vi "VISJS Viewer.vi"(4 "Extra Scripts":string, 5 "FileDependency out":map{path, T1}(c390), 6 "Options":string, 7 "OpenWebBrowser(False)":bool, 8 "error in":errorcluster, 9 "Embedd VISJS Librarya in HTMl File(False)":bool, 10 "HTMLFilePath":path, 11 "LibraryDependency":map{path, T3}(c390)) -> (0 "error out":errorcluster, 3 "HTMLFileContent":string)   [LabVIEW 2020, in "VISJS Viewer.lvlib"] (continued)
this.evTarget,this.domHandler),this.evWin&&Bp(Sp(this.element),this.evWin,this.domHandler)},t.destroy=function(){this.evEl&&zp(this.element,this.evEl,this.domHandler),this.evTarget&&zp(this.target,this.evTarget,this.domHandler),this.evWin&&zp(Sp(this.element),this.evWin,this.domHandler)},g}();function Fp(g,t,A){if(g.indexOf&&!A)return g.indexOf(t);for(var e=0;e<g.length;){if(A&&g[e][A]==t||!A&&g[e]===t)return e;e++}return-1}var Gp={pointerdown:op,pointermove:2,pointerup:np,pointercancel:rp,pointerout:rp},jp={2:Cp,3:\"pen\",4:Ip,5:\"kinect\"},Lp=\"pointerdown\",Vp=\"pointermove pointerup pointercancel\";Fu.MSPointerEvent&&!Fu.PointerEvent&&(Lp=\"MSPointerDown\",Vp=\"MSPointerMove MSPointerUp MSPointerCancel\");var Yp=function(g){function t(){var A,e=t.prototype;return e.evEl=Lp,e.evWin=Vp,(A=g.apply(this,arguments)||this).store=A.manager.session.pointerEvents=[],A}return Su(t,g),t.prototype.handler=function(g){var t=this.store,A=!1,e=g.type.toLowerCase().replace(\"ms\",\"\"),C=Gp[e],I=jp[g.pointerType]||g.pointerType,i=I===Cp,o=Fp(t,g.pointerId,\"pointerId\");C&op&&(0===g.button||i)?o<0&&(t.push(g),o=t.length-1):C&(np|rp)&&(A=!0),o<0||(t[o]=g,this.callback(this.manager,C,{pointers:t,changedPointers:[g],pointerType:I,srcEvent:g}),A&&t.splice(o,1))},t}(Zp);function Wp(g){return Array.prototype.slice.call(g,0)}function Qp(g,t,A){for(var e=[],C=[],I=0;I<g.length;){var i=t?g[I][t]:g[I];Fp(C,i)<0&&e.push(g[I]),C[I]=i,I++}return A&&(e=t?e.sort((function(g,A){return g[t]>A[t]})):e.sort()),e}var Up={touchstart:op,touchmove:2,touchend:np,touchcancel:rp},_p=function(g){function t(){var A;return t.prototype.evTarget=\"touchstart touchmove touchend touchcancel\",(A=g.apply(this,arguments)||this).targetIds={},A}return Su(t,g),t.prototype.handler=function(g){var t=Up[g.type],A=Kp.call(this,g,t);A&&this.callback(this.manager,t,{pointers:A[0],changedPointers:A[1],pointerType:Cp,srcEvent:g})},t}(Zp);function Kp(g,t){var A,e,C=Wp(g.touches),I=this.targetIds;if(t&(2|op)&&1===C.length)return I[C[0].identifier]=!0,[C,C];var i=Wp(g.changedTouches),o=[],n=this.target;if(e=C.filter((function(g){return kp(g.target,n)})),t===op)for(A=0;A<e.length;)I[e[A].identifier]=!0,A++;for(A=0;A<i.length;)I[i[A].identifier]&&o.push(i[A]),t&(np|rp)&&delete I[i[A].identifier],A++;return o.length?[Qp(e.concat(o),\"identifier\",!0),o]:void 0}var Hp={mousedown:op,mousemove:2,mouseup:np},Xp=function(g){function t(){var A,e=t.prototype;return e.evEl=\"mousedown\",e.evWin=\"mousemove mouseup\",(A=g.apply(this,arguments)||this).pressed=!1,A}return Su(t,g),t.prototype.handler=function(g){var t=Hp[g.type];t&op&&0===g.button&&(this.pressed=!0),2&t&&1!==g.which&&(t=np),this.pressed&&(t&np&&(this.pressed=!1),this.callback(this.manager,t,{pointers:[g],changedPointers:[g],pointerType:Ip,srcEvent:g}))},t}(Zp),Jp=2500;function qp(g){var t=g.changedPointers[0];if(t.identifier===this.primaryTouch){var A={x:t.clientX,y:t.clientY},e=this.lastTouches;this.lastTouches.push(A);setTimeout((function(){var g=e.indexOf(A);g>-1&&e.splice(g,1)}),Jp)}}function $p(g,t){g&op?(this.primaryTouch=t.changedPointers[0].identifier,qp.call(this,t)):g&(np|rp)&&qp.call(this,t)}function gf(g){for(var t=g.srcEvent.clientX,A=g.srcEvent.clientY,e=0;e<this.lastTouches.length;e++){var C=this.lastTouches[e],I=Math.abs(t-C.x),i=Math.abs(A-C.y);if(I<=25&&i<=25)return!0}return!1}var tf=function(){return function(g){function t(t,A){var e;return(e=g.call(this,t,A)||this).handler=function(g,t,A){var C=A.pointerType===Cp,I=A.pointerType===Ip;if(!(I&&A.sourceCapabilities&&A.sourceCapabilities.firesTouchEvents)){if(C)$p.call(Zu(Zu(e)),t,A);else if(I&&gf.call(Zu(Zu(e)),A))return;e.callback(g,t,A)}},e.touch=new _p(e.manager,e.handler),e.mouse=new Xp(e.manager,e.handler),e.primaryTouch=null,e.lastTouches=[],e}return Su(t,g),t.prototype.destroy=function(){this.touch.destroy(),this.mouse.destroy()},t}(Zp)}();function Af(g,t,A){return!!Array.isArray(g)&&(yp(g,A[t],A),!0)}var ef=32,Cf=1;function If(g,t){var A=t.manager;return A?A.get(g):g}function of(g){return 16&g?\"cancel\":8&g?\"end\":4&g?\"move\":2&g?\"start\":\"\"}var nf=function(){function g(g){void 0===g&&(g={}),this.options=zu({enable:!0},g),this.id=Cf++,this.manager=null,this.state=1,this.simultaneous={},this.requireFail=[]}var t=g.prototype;return t.set=function(g){return Gu(this.options,g),this.manager&&this.manager.touchAction.update(),this},t.recognizeWith=function(g){if(Af(g,\"recognizeWith\",this))return this;var t=this.simultaneous;return t[(g=If(g,this)).id]||(t[g.id]=g,g.recognizeWith(this)),this},t.dropRecognizeWith=function(g){return Af(g,\"dropRecognizeWith\",this)||(g=If(g,this),delete this.simultaneous[g.id]),this},t.requireFailure=function(g){if(Af(g,\"requireFailure\",this))return this;var t=this.requireFail;return-1===Fp(t,g=If(g,this))&&(t.push(g),g.requireFailure(this)),this},t.dropRequireFailure=function(g){if(Af(g,\"dropRequireFailure\",this))return this;g=If(g,this);var t=Fp(this.requireFail,g);return t>-1&&this.requireFail.splice(t,1),this},t.hasRequireFailures=function(){return this.requireFail.length>0},t.canRecognizeWith=function(g){return!!this.simultaneous[g.id]},t.emit=function(g){var t=this,A=this.state;function e(A){t.manager.emit(A,g)}A<8&&e(t.options.event+of(A)),e(t.options.event),g.additionalEvent&&e(g.additionalEvent),A>=8&&e(t.options.event+of(A))},t.tryEmit=function(g){if(this.canEmit())return this.emit(g);this.state=ef},t.canEmit=function(){for(var g=0;g<this.requireFail.length;){if(!(33&this.requireFail[g].state))return!1;g++}return!0},t.recognize=function(g){var t=Gu({},g);if(!mp(this.options.enable,[this,t]))return this.reset(),void(this.state=ef);56&this.state&&(this.state=1),this.state=this.process(t),30&this.state&&this.tryEmit(t)},t.process=function(g){},t.getTouchAction=function(){},t.reset=function(){},g}(),rf=function(g){function t(t){var A;return void 0===t&&(t={}),(A=g.call(this,zu({event:\"tap\",pointers:1,taps:1,interval:300,time:250,threshold:9,posThreshold:10},t))||this).pTime=!1,A.pCenter=!1,A._timer=null,A._input=null,A.count=0,A}Su(t,g);var A=t.prototype;return A.getTouchAction=function(){return[Xu]},A.process=function(g){var t=this,A=this.options,e=g.pointers.length===A.pointers,C=g.distance<A.threshold,I=g.deltaTime<A.time;if(this.reset(),g.eventType&op&&0===this.count)return this.failTimeout();if(C&&I&&e){if(g.eventType!==np)return this.failTimeout();var i=!this.pTime||g.timeStamp-this.pTime<A.interval,o=!this.pCenter||Op(this.pCenter,g.center)<A.posThreshold;if(this.pTime=g.timeStamp,this.pCenter=g.center,o&&i?this.count+=1:this.count=1,this._input=g,0===this.count%A.taps)return this.hasRequireFailures()?(this._timer=setTimeout((function(){t.state=8,t.tryEmit()}),A.interval),2):8}return ef},A.failTimeout=function(){var g=this;return this._timer=setTimeout((function(){g.state=ef}),this.options.interval),ef},A.reset=function(){clearTimeout(this._timer)},A.emit=function(){8===this.state&&(this._input.tapCount=this.count,this.manager.emit(this.options.event,this._input))},t}(nf),sf=function(g){function t(t){return void 0===t&&(t={}),g.call(this,zu({pointers:1},t))||this}Su(t,g);var A=t.prototype;return A.attrTest=function(g){var t=this.options.pointers;return 0===t||g.pointers.length===t},A.process=function(g){var t=this.state,A=g.eventType,e=6&t,C=this.attrTest(g);return e&&(A&rp||!C)?16|t:e||C?A&np?8|t:2&t?4|t:2:ef},t}(nf);function af(g){return g===lp?\"down\":g===hp?\"up\":g===ap?\"left\":g===dp?\"right\":\"\"}var df=function(g){function t(t){var A;return void 0===t&&(t={}),(A=g.call(this,zu({event:\"pan\",threshold:10,pointers:1,direction:pp},t))||this).pX=null,A.pY=null,A}Su(t,g);var A=t.prototype;return A.getTouchAction=function(){var g=this.options.direction,t=[];return g&cp&&t.push($u),g&up&&t.push(qu),t},A.directionTest=function(g){var t=this.options,A=!0,e=g.distance,C=g.direction,I=g.deltaX,i=g.deltaY;return C&t.direction||(t.direction&cp?(C=0===I?sp:I<0?ap:dp,A=I!==this.pX,e=Math.abs(g.deltaX)):(C=0===i?sp:i<0?hp:lp,A=i!==this.pY,e=Math.abs(g.deltaY))),g.direction=C,A&&e>t.threshold&&C&t.direction},A.attrTest=function(g){return sf.prototype.attrTest.call(this,g)&&(2&this.state||!(2&this.state)&&this.directionTest(g))},A.emit=function(t){this.pX=t.deltaX,this.pY=t.deltaY;var A=af(t.direction);A&&(t.additionalEvent=this.options.event+A),g.prototype.emit.call(this,t)},t}(sf),hf=function(g){function t(t){return void 0===t&&(t={}),g.call(this,zu({event:\"swipe\",threshold:10,velocity:.3,direction:cp|up,pointers:1},t))||this}Su(t,g);var A=t.prototype;return A.getTouchAction=function(){return df.prototype.getTouchAction.call(this)},A.attrTest=function(t){var A,e=this.options.direction;return e&(cp|up)?A=t.overallVelocity:e&cp?A=t.overallVelocityX:e&up&&(A=t.overallVelocityY),g.prototype.attrTest.call(this,t)&&e&t.offsetDirection&&t.distance>this.options.threshold&&t.maxPointers===this.options.pointers&&Yu(A)>this.options.velocity&&t.eventType&np},A.emit=function(g){var t=af(g.offsetDirection);t&&this.manager.emit(this.options.event+t,g),this.manager.emit(this.options.event,g)},t}(sf),lf=function(g){function t(t){return void 0===t&&(t={}),g.call(this,zu({event:\"pinch\",threshold:0,pointers:2},t))||this}Su(t,g);var A=t.prototype;return A.getTouchAction=function(){return[Ju]},A.attrTest=function(t){return g.prototype.attrTest.call(this,t)&&(Math.abs(t.scale-1)>this.options.threshold||2&this.state)},A.emit=function(t){if(1!==t.scale){var A=t.scale<1?\"in\":\"out\";t.additionalEvent=this.options.event+A}g.prototype.emit.call(this,t)},t}(sf),cf=function(g){function t(t){return void 0===t&&(t={}),g.call(this,zu({event:\"rotate\",threshold:0,pointers:2},t))||this}Su(t,g);var A=t.prototype;return A.getTouchAction=function(){return[Ju]},A.attrTest=function(t){return g.prototype.attrTest.call(this,t)&&(Math.abs(t.rotation)>this.options.threshold||2&this.state)},t}(sf),uf=function(g){function t(t){var A;return void 0===t&&(t={}),(A=g.call(this,zu({event:\"press\",pointers:1,time:251,threshold:9},t))||this)._timer=null,A._input=null,A}Su(t,g);var A=t.prototype;return A.getTouchAction=function(){return[Hu]},A.process=function(g){var t=this,A=this.options,e=g.pointers.length===A.pointers,C=g.distance<A.threshold,I=g.deltaTime>A.time;if(this._input=g,!C||!e||g.eventType&(np|rp)&&!I)this.reset();else if(g.eventType&op)this.reset(),this._timer=setTimeout((function(){t.state=8,t.tryEmit()}),A.time);else if(g.eventType&np)return 8;return ef},A.reset=function(){clearTimeout(this._timer)},A.emit=function(g){8===this.state&&(g&&g.eventType&np?this.manager.emit(this.options.event+\"up\",g):(this._input.timeStamp=Wu(),this.manager.emit(this.options.event,this._input)))},t}(nf),pf={domEvents:!1,touchAction:Ku,enable:!0,inputTarget:null,inputClass:null,cssProps:{userSelect:\"none\",touchSelect:\"none\",touchCallout:\"none\",contentZooming:\"none\",userDrag:\"none\",tapHighlightColor:\"rgba(0,0,0,0)\"}},ff=[[cf,{enable:!1}],[lf,{enable:!1},[\"rotate\"]],[hf,{direction:cp}],[df,{direction:cp},[\"swipe\"]],[rf],[rf,{event:\"doubletap\",taps:2},[\"tap\"]],[uf]];function vf(g,t){var A,e=g.element;e.style&&(yp(g.options.cssProps,(function(C,I){A=Qu(e.style,I),t?(g.oldCssProps[A]=e.style[A],e.style[A]=C):e.style[A]=g.oldCssProps[A]||\"\"})),t||(g.oldCssProps={}))}var yf=function(){function g(g,t){var A,e=this;this.options=Gu({},pf,t||{}),this.options.inputTarget=this.options.inputTarget||g,this.handlers={},this.session={},this.recognizers=[],this.oldCssProps={},this.element=g,this.input=new((A=this).options.inputClass||(Ap?Yp:ep?_p:tp?tf:Xp))(A,Pp),this.touchAction=new wp(this,this.options.touchAction),vf(this,!0),yp(this.options.recognizers,(function(g){var t=e.add(new g[0](g[1]));g[2]&&t.recognizeWith(g[2]),g[3]&&t.requireFailure(g[3])}),this)}var t=g.prototype;return t.set=function(g){return Gu(this.options,g),g.touchAction&&this.touchAction.update(),g.inputTarget&&(this.input.destroy(),this.input.target=g.inputTarget,this.input.init()),this},t.stop=function(g){this.session.stopped=g?2:1},t.recognize=function(g){var t=this.session;if(!t.stopped){var A;this.touchAction.preventDefaults(g);var e=this.recognizers,C=t.curRecognizer;(!C||C&&8&C.state)&&(t.curRecognizer=null,C=null);for(var I=0;I<e.length;)A=e[I],2===t.stopped||C&&A!==C&&!A.canRecognizeWith(C)?A.reset():A.recognize(g),!C&&14&A.state&&(t.curRecognizer=A,C=A),I++}},t.get=function(g){if(g instanceof nf)return g;for(var t=this.recognizers,A=0;A<t.length;A++)if(t[A].options.event===g)return t[A];return null},t.add=function(g){if(Af(g,\"add\",this))return this;var t=this.get(g.options.event);return t&&this.remove(t),this.recognizers.push(g),g.manager=this,this.touchAction.update(),g},t.remove=function(g){if(Af(g,\"remove\",this))return this;var t=this.get(g);if(g){var A=this.recognizers,e=Fp(A,t);-1!==e&&(A.splice(e,1),this.touchAction.update())}return this},t.on=function(g,t){if(void 0===g||void 0===t)return this;var A=this.handlers;return yp(Mp(g),(function(g){A[g]=A[g]||[],A[g].push(t)})),this},t.off=function(g,t){if(void 0===g)return this;var A=this.handlers;return yp(Mp(g),(function(g){t?A[g]&&A[g].splice(Fp(A[g],t),1):delete A[g]})),this},t.emit=function(g,t){this.options.domEvents&&function(g,t){var A=document.createEvent(\"Event\");A.initEvent(g,!0,!0),A.gesture=t,t.target.dispatchEvent(A)}(g,t);var A=this.handlers[g]&&this.handlers[g].slice();if(A&&A.length){t.type=g,t.preventDefault=function(){t.srcEvent.preventDefault()};for(var e=0;e<A.length;)A[e](t),e++}},t.destroy=function(){this.element&&vf(this,!1),this.handlers={},this.session={},this.input.destroy(),this.element=null},g}(),mf={touchstart:op,touchmove:2,touchend:np,touchcancel:rp},bf=function(g){function t(){var A,e=t.prototype;return e.evTarget=\"touchstart\",e.evWin=\"touchstart touchmove touchend touchcancel\",(A=g.apply(this,arguments)||this).started=!1,A}return Su(t,g),t.prototype.handler=function(g){var t=mf[g.type];if(t===op&&(this.started=!0),this.started){var A=wf.call(this,g,t);t&(np|rp)&&A[0].length-A[1].length==0&&(this.started=!1),this.callback(this.manager,t,{pointers:A[0],changedPointers:A[1],pointerType:Cp,srcEvent:g})}},t}(Zp);function wf(g,t){var A=Wp(g.touches),e=Wp(g.changedTouches);return t&(np|rp)&&(A=Qp(A.concat(e),\"identifier\",!0)),[A,e]}function kf(g,t,A){var e=\"DEPRECATED METHOD: \"+t+\"\\n\"+A+\" AT \\n\";return function(){var t=new Error(\"get-stack-trace\"),A=t&&t.stack?t.stack.replace(/^[^\\(]+?[\\n$]/gm,\"\").replace(/^\\s+at\\s+/gm,\"\").replace(/^Object.<anonymous>\\s*\\(/gm,\"{anonymous}()@\"):\"Unknown Stack Trace\",C=window.console&&(window.console.warn||window.console.log);return C&&C.call(window.console,e,A),g.apply(this,arguments)}}var xf=kf((function(g,t,A){for(var e=Object.keys(t),C=0;C<e.length;)(!A||A&&void 0===g[e[C]])&&(g[e[C]]=t[e[C]]),C++;return g}),\"extend\",\"Use `assign`.\"),Ef=kf((function(g,t){return xf(g,t,!0)}),\"merge\",\"Use `assign`.\");function Of(g,t,A){var e,C=t.prototype;(e=g.prototype=Object.create(C)).constructor=g,e._super=C,A&&Gu(e,A)}function Tf(g,t){return function(){return g.apply(t,arguments)}}var Df=function(){var g=function(g,t){return void 0===t&&(t={}),new yf(g,zu({recognizers:ff.concat()},t))};return g.VERSION=\"2.0.17-rc\",g.DIRECTION_ALL=pp,g.DIRECTION_DOWN=lp,g.DIRECTION_LEFT=ap,g.DIRECTION_RIGHT=dp,g.DIRECTION_UP=hp,g.DIRECTION_HORIZONTAL=cp,g.DIRECTION_VERTICAL=up,g.DIRECTION_NONE=sp,g.DIRECTION_DOWN=lp,g.INPUT_START=op,g.INPUT_MOVE=2,g.INPUT_END=np,g.INPUT_CANCEL=rp,g.STATE_POSSIBLE=1,g.STATE_BEGAN=2,g.STATE_CHANGED=4,g.STATE_ENDED=8,g.STATE_RECOGNIZED=8,g.STATE_CANCELLED=16,g.STATE_FAILED=ef,g.Manager=yf,g.Input=Zp,g.TouchAction=wp,g.TouchInput=_p,g.MouseInput=Xp,g.PointerEventInput=Yp,g.TouchMouseInput=tf,g.SingleTouchInput=bf,g.Recognizer=nf,g.AttrRecognizer=sf,g.Tap=rf,g.Pan=df,g.Swipe=hf,g.Pinch=lf,g.Rotate=cf,g.Press=uf,g.on=Bp,g.off=zp,g.each=yp,g.merge=Ef,g.extend=xf,g.bindFn=Tf,g.assign=Gu,g.inherit=Of,g.bindFn=Tf,g.prefixed=Qu,g.toArray=Wp,g.inArray=Fp,g.uniqueArray=Qp,g.splitStr=Mp,g.boolOrFn=mp,g.hasParent=kp,g.addEventListeners=Bp,g.removeEventListeners=zp,g.defaults=Gu({},pf,{preset:ff}),g}();Df.defaults;var Nf=Df;function Rf(g,t){var A=void 0!==uh&&ln(g)||g[\"@@iterator\"];if(!A){if(Rh(g)||(A=function(g,t){var A;if(!g)return;if(\"string\"==typeof g)return Pf(g,t);var e=wh(A=Object.prototype.toString.call(g)).call(A,8,-1);\"Object\"===e&&g.constructor&&(e=g.constructor.name);if(\"Map\"===e||\"Set\"===e)return Uo(g);if(\"Arguments\"===e||/^(?:Ui|I)nt(?:8|16|32)(?:Clamped)?Array$/.test(e))return Pf(g,t)}(g))||t&&g&&\"number\"==typeof g.length){A&&(g=A);var e=0,C=function(){};return{s:C,n:function(){return e>=g.length?{done:!0}:{done:!1,value:g[e++]}},e:function(g){throw g},f:C}}throw new TypeError(\"Invalid attempt to iterate non-iterable instance.\\nIn order to be iterable, non-array objects must have a [Symbol.iterator]() method.\")}var I,i=!0,o=!1;return{s:function(){A=A.call(g)},n:function(){var g=A.next();return i=g.done,g},e:function(g){o=!0,I=g},f:function(){try{i||null==A.return||A.return()}finally{if(o)throw I}}}}function Pf(g,t){(null==t||t>g.length)&&(t=g.length);for(var A=0,e=new Array(t);A<t;A++)e[A]=g[A];return e}var Mf=uh(\"DELETE\");function Bf(){var g=zf.apply(void 0,arguments);return Zf(g),g}function zf(){for(var g=arguments.length,t=new Array(g),A=0;A<g;A++)t[A]=arguments[A];if(t.length<2)return t[0];var e;if(t.length>2)return zf.apply(void 0,bh(e=[Bf(t[0],t[1])]).call(e,ch(wh(t).call(t,2))));var C=t[0],I=t[1];if(C instanceof Date&&I instanceof Date)return C.setTime(I.getTime()),C;var i,o=Rf(Nh(I));try{for(o.s();!(i=o.n()).done;){var n=i.value;Object.prototype.propertyIsEnumerable.call(I,n)&&(I[n]===Mf?delete C[n]:null===C[n]||null===I[n]||\"object\"!==yd(C[n])||\"object\"!==yd(I[n])||Rh(C[n])||Rh(I[n])?C[n]=Sf(I[n]):C[n]=zf(C[n],I[n]))}}catch(g){o.e(g)}finally{o.f()}return C}function Sf(g){return Rh(g)?Fh(g).call(g,(function(g){return Sf(g)})):\"object\"===yd(g)&&null!==g?g instanceof Date?new Date(g.getTime()):zf({},g):g}function Zf(g){for(var t=0,A=Lh(g);t<A.length;t++){var e=A[t];g[e]===Mf?delete g[e]:\"object\"===yd(g[e])&&null!==g[e]&&Zf(g[e])}}function Ff(){for(var g=arguments.length,t=new Array(g),A=0;A<g;A++)t[A]=arguments[A];return function(g){var t=function(){for(var g=function(){var g=4022871197;return function(t){for(var A=t.toString(),e=0;e<A.length;e++){var C=.02519603282416938*(g+=A.charCodeAt(e));C-=g=C>>>0,g=(C*=g)>>>0,g+=4294967296*(C-=g)}return 2.3283064365386963e-10*(g>>>0)}}(),t=g(\" \"),A=g(\" \"),e=g(\" \"),C=0;C<arguments.length;C++)(t-=g(C<0||arguments.length<=C?void 0:arguments[C]))<0&&(t+=1),(A-=g(C<0||arguments.length<=C?void 0:arguments[C]))<0&&(A+=1),(e-=g(C<0||arguments.length<=C?void 0:arguments[C]))<0&&(e+=1);return[t,A,e]}(g),A=lh(t,3),e=A[0],C=A[1],I=A[2],i=1,o=function(){var g=2091639*e+2.3283064365386963e-10*i;return e=C,C=I,I=g-(i=0|g)};return o.uint32=function(){return 4294967296*o()},o.fract53=function(){return o()+11102230246251565e-32*(2097152*o()|0)},o.algorithm=\"Alea\",o.seed=g,o.version=\"0.9\",o}(t.length?t:[Qh()])}var Gf=\"undefined\"!=typeof window?window.Hammer||Nf:function(){return function(){var g=function(){};return{on:g,off:g,destroy:g,emit:g,get:function(){return{set:g}}}}()};function jf(g){var t,A=this;this._cleanupQueue=[],this.active=!1,this._dom={container:g,overlay:document.createElement(\"div\")},this._dom.overlay.classList.add(\"vis-overlay\"),this._dom.container.appendChild(this._dom.overlay),this._cleanupQueue.push((function(){A._dom.overlay.parentNode.removeChild(A._dom.overlay)}));var e=Gf(this._dom.overlay);e.on(\"tap\",je(t=this._onTapOverlay).call(t,this)),this._cleanupQueue.push((function(){e.destroy()}));var C=[\"tap\",\"doubletap\",\"press\",\"pinch\",\"pan\",\"panstart\",\"panmove\",\"panend\"];Cl(C).call(C,(function(g){e.on(g,(function(g){g.srcEvent.stopPropagation()}))})),document&&document.body&&(this._onClick=function(t){(function(g,t){for(;g;){if(g===t)return!0;g=g.parentNode}return!1})(t.target
